vi "Units_RadiansPerSecondToRotationsPerMinute.vi"(10 "RadiansPerSecond":dbl) -> (2 "RotationsPerMinute":dbl)   [LabVIEW 2019, in "Trajectory_Library.lvlib"]
doc: "Convert a value from radians/sec to revolutions per minute (RPM)\n\nInputs: \n - RadiansPerSec - Speed (Radians / Second)\n\nOutputs:\n - RevolutionsPerMinute - Speed ( RPM )"
uses:
  Trajectory_Library.lvlib
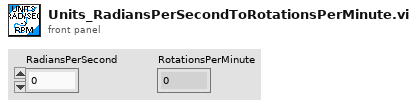
[diagram p1: front panel]
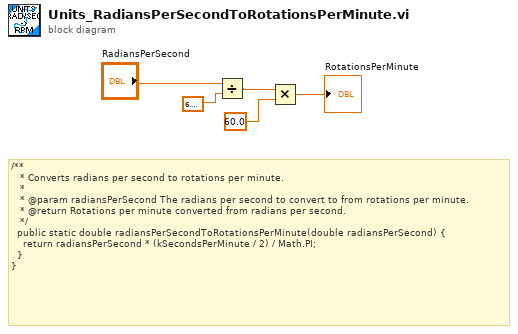
[diagram p0: block diagram]
diagram:
  # "/**\n   * Converts radians per second to rotations per minute.\n   *\n   * @param radiansPerSecond The radians per second to convert to from rotations per minute.\n   * @return Rotations per minute converted from radians per second.\n   */\n  public static double radiansPerSecondToRotationsPerMinute(double radiansPerSecond) {\n    return radiansPerSecond * (kSecondsPerMinute / 2) / Math.PI;\n  }\n}"
  n1 = Divide(x="RadiansPerSecond", y=6.283185307179586) -> (x/y=w2:dbl)
  n2 = Multiply(x=w2, y=60.0) -> (x*y=→"RotationsPerMinute":dbl)
